vi "Ex5_ForLoop.vi"() -> ()   [LabVIEW 2024]
panel:
  out "Array":dbl[](array[numeric])
  out "Numeric":i32
  out "number (0 to 1)":dbl
  in  "Numeric 2":i32
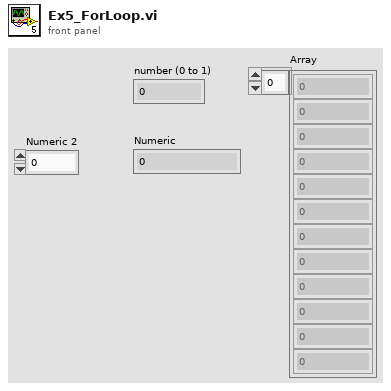
[diagram p1: front panel]
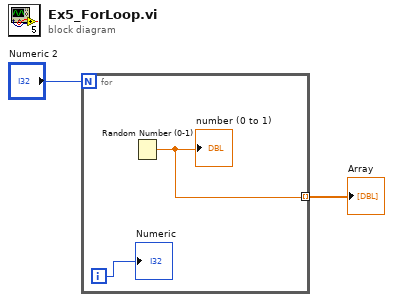
[diagram p0: block diagram]
diagram:
  n1 = for {
    N: "Numeric 2" -> [_]
    tunnel: [w3] -> w1 mode=indexing
    i -> [w4]
    n2 = Random Number (0-1)() -> (number: 0 to 1=w3:dbl)
    "number (0 to 1)" <- w3
    "Numeric" <- w4
  }
  "Array" <- w1
